vi "Save File DOE Get Program Info.vi"(10 "LV Program":T1=enum."DOE Stand", 11 "File Paths":T2={"General Setup Paths"={"Calibration File Path"=path "C:/Program Files/GE/Washer DOE/CalibrationDates.txt", "DOE Capacity Path"=path "C:/Program Files/GE/Washer DOE/DOE Capacity.txt", "Data Folder Path"=path "C:/Program Files/GE/Washer DOE/CalibrationDates.txt", "RLT Backup Data Path"=path "C:/Program Files/GE/Washer DOE/CalibrationDates.txt", "Tool Base Path"=path "C:/Program Files/GE/Washer DOE/CalibrationDates.txt", "General Startup Config Path"=path "C:/Program Files/GE/Washer DOE/CalibrationDates.txt", "File Save Previous Run Path"=path "", "File Save Configuration Data Path"=path ""}, "Data File Paths"={"Data File Path"=path "", "Debug File Path"=path "", "Bus Log Path"=path "", "Current"=path "", "Summary"=path ""}, "New Summary Created"=FALSE, "Check Location Interval (Second)"=0}) -> (1 "Headers":string[](array[string]), 2 "Model Information":string[][](array[string]), 3 "Program Names":string[](array[string]))   [LabVIEW 2016, in "File Setup.lvlib"]
uses:
  File Setup.lvlib
  File Setup (Public)/Type Definition/Save File DOE File Path Control.ctl
  File Setup (Public)/Type Definition/Save File DOE LabView Program.ctl
  File Setup (Public)/Type Definition/Save File DOE Data Save Filepaths.ctl
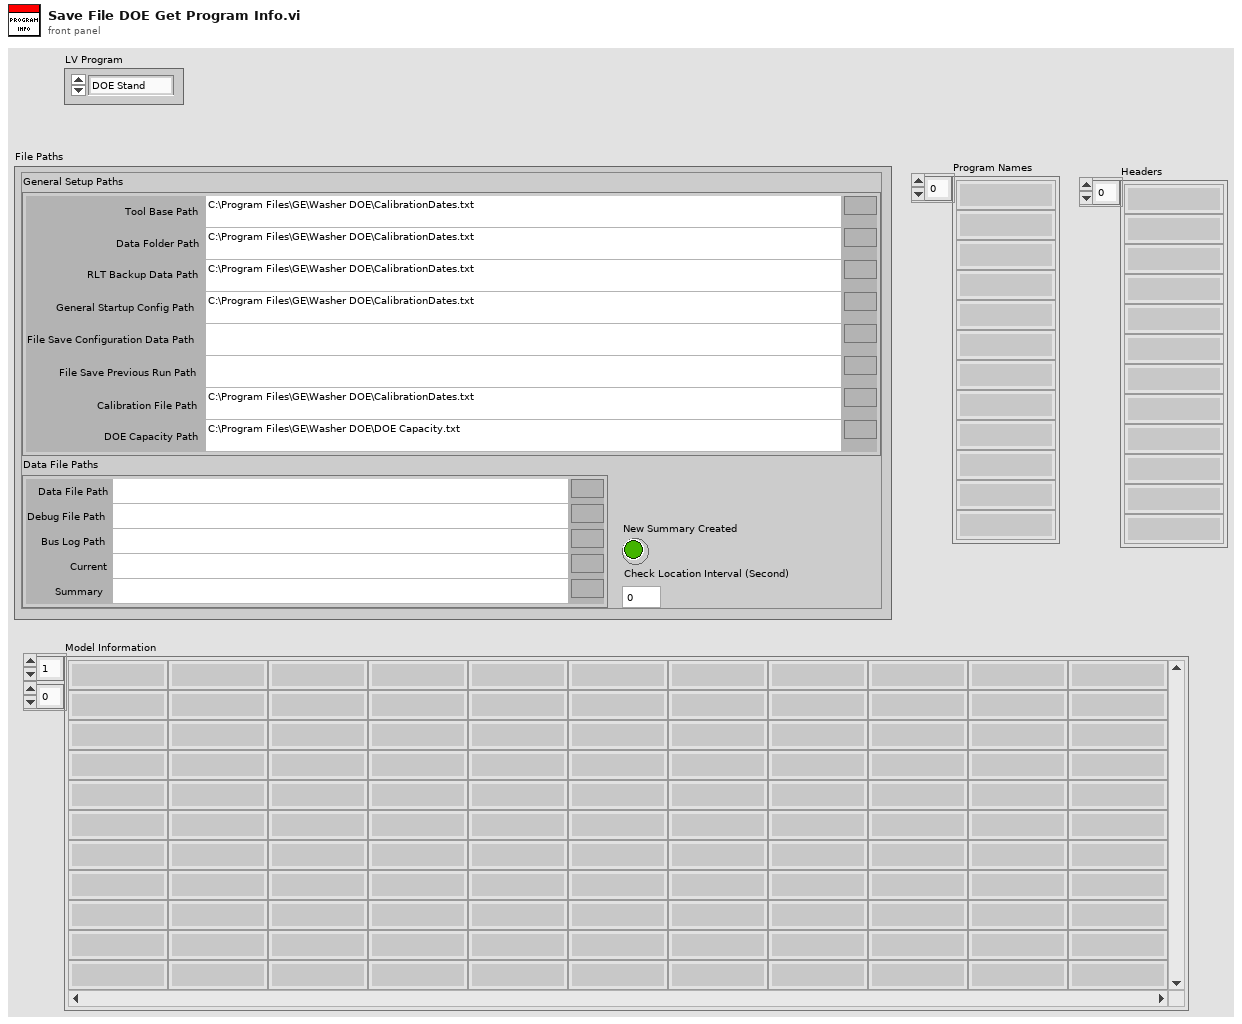
[diagram p1: front panel]
types:
  T1 = typedef "File Setup.lvlib/Save File DOE LabView Program.ctl" = enum16{"No Name Found", "DOE Stand", "Dishwasher Kitchen", "Portable Stand", "HEWH", "Dryer", "Dryer WILT", "HCC", "PRAT", "HEWH RLT"}
  T2 = typedef "File Setup.lvlib/Save File DOE File Path Control.ctl" = cluster{"General Setup Paths":cluster{"Calibration File Path":path, "DOE Capacity Path":path, "Data Folder Path":path, "RLT Backup Data Path":path, "Tool Base Path":path, "General Startup Config Path":path, "File Save Previous Run Path":path, "File Save Configuration Data Path":path}, "Data File Paths":T3, "New Summary Created":bool, "Check Location Interval (Second)":i32}
  T3 = typedef "File Setup.lvlib/Save File DOE Data Save Filepaths.ctl" = cluster{"Data File Path":path, "Debug File Path":path, "Bus Log Path":path, "Current":path, "Summary":path}
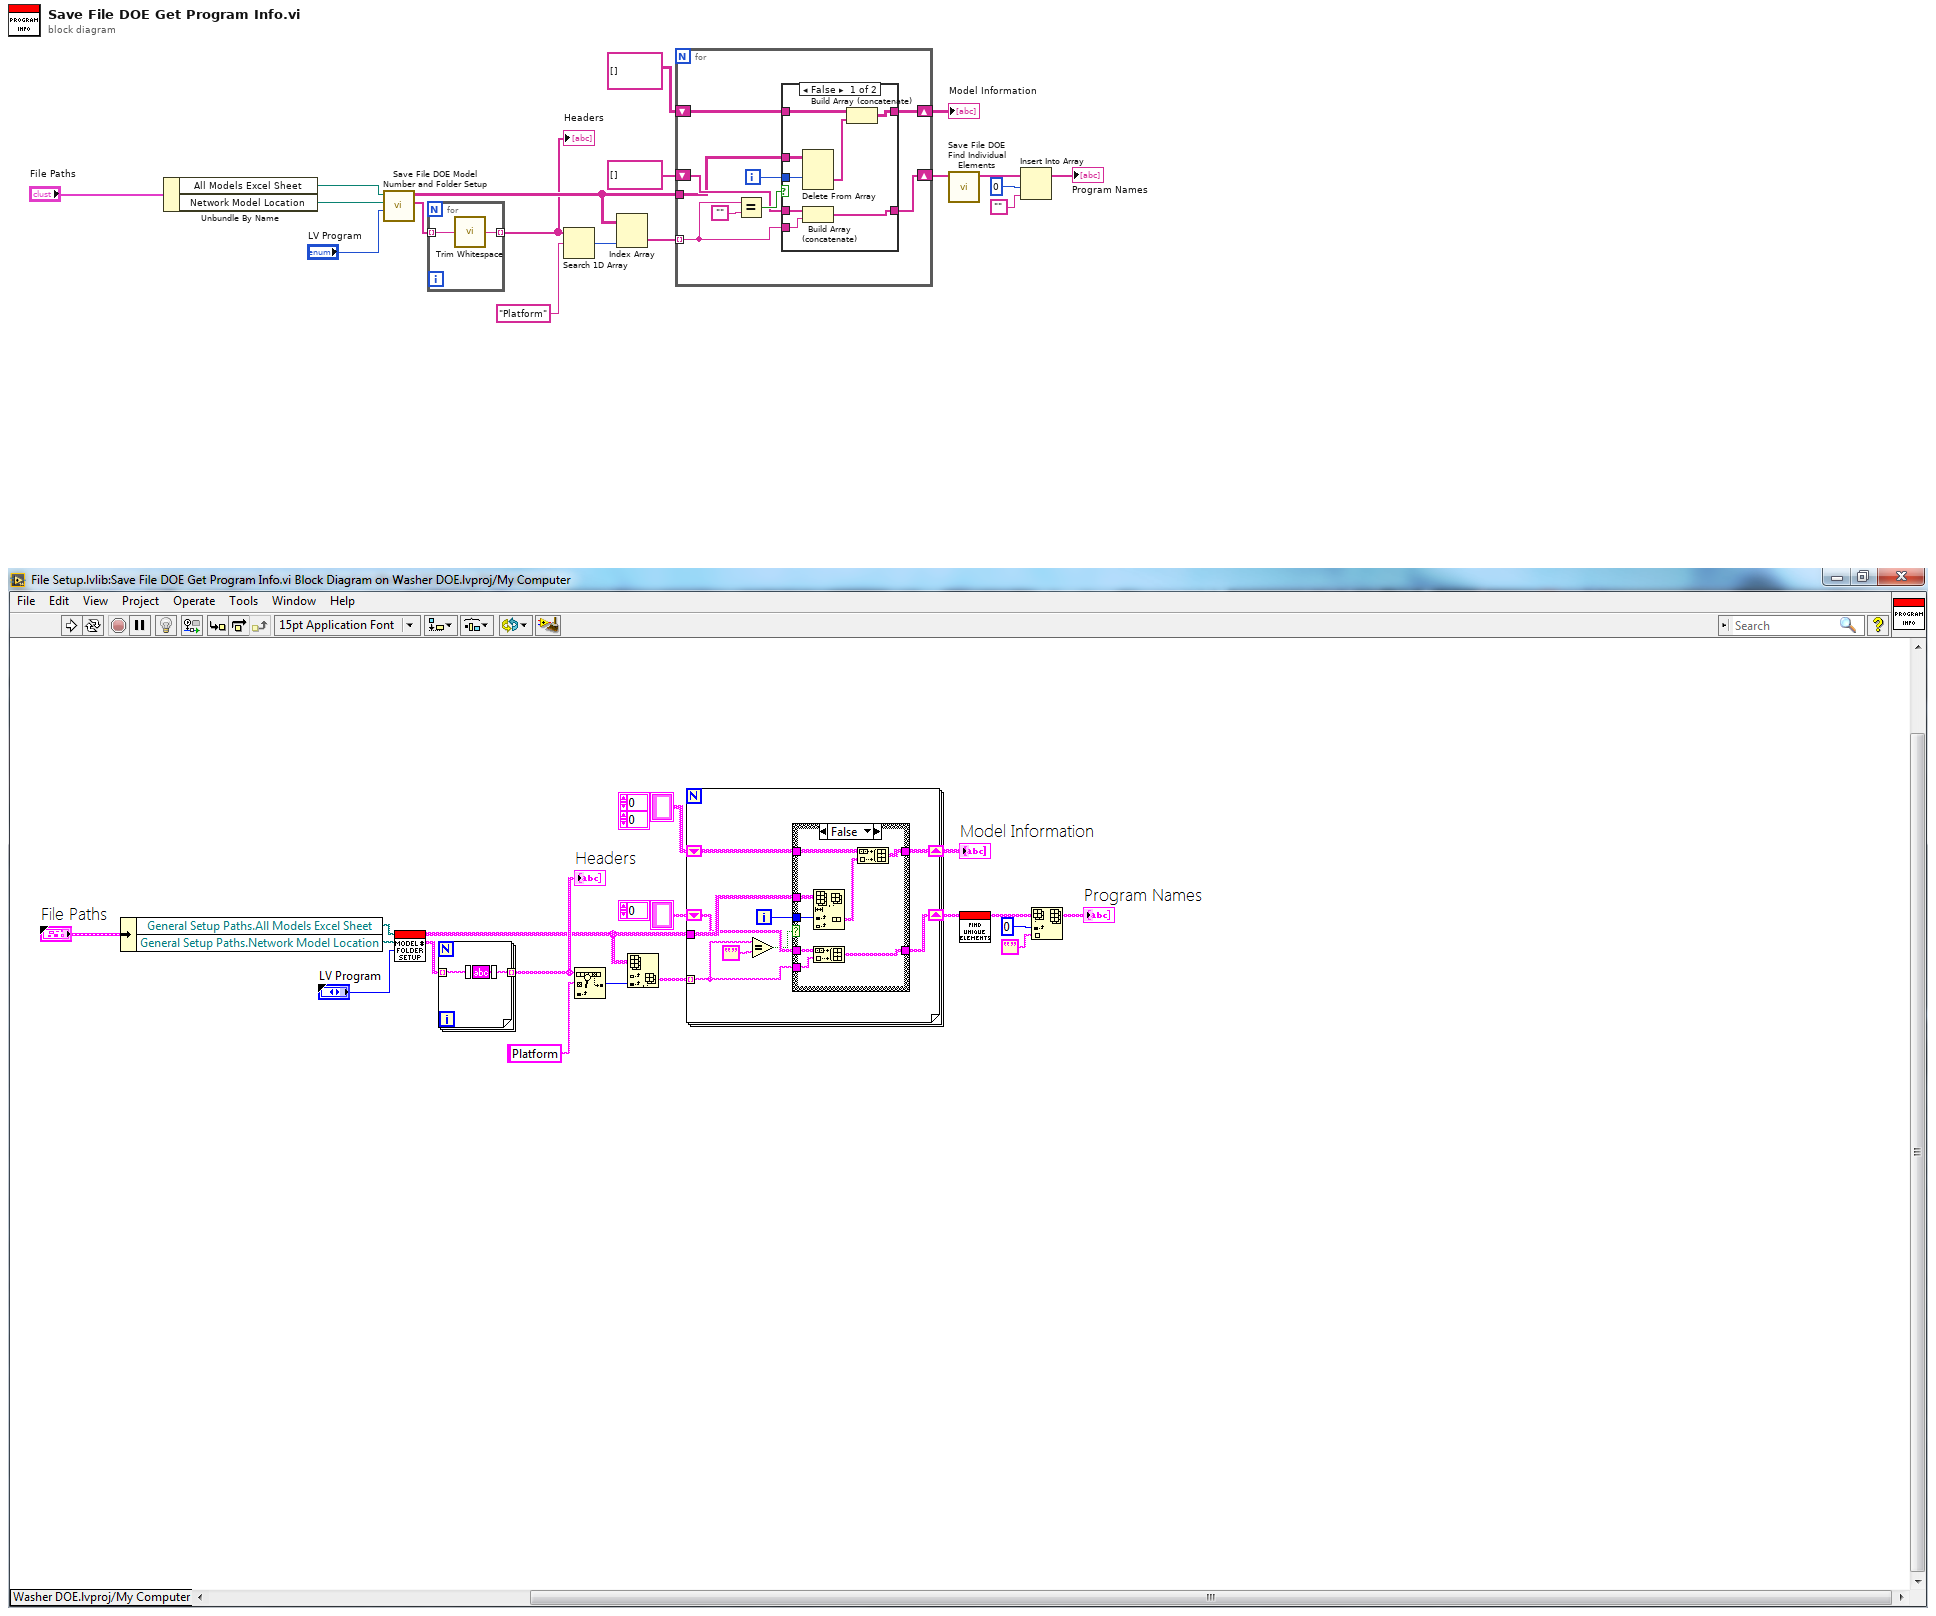
[diagram p0: block diagram]
diagram:
  n1 = Unbundle By Name("File Paths") -> ("All Models Excel Sheet"=w9:path, "Network Model Location"=w10:path)
  n2 = call "Save File DOE Model Number and Folder Setup.vi"("LV Program"="LV Program", "Network Model Location"=w10, "All Models Excel Sheet"=w9) -> ("Header"=w18:string[], "Model Data"=w15:string[][])  [unwired: 7 in]
  n3 = for {
    tunnel: w18 -> [w20] mode=indexing
    tunnel: [w19] -> w4 mode=indexing
    n4 = call <vilib>:"Trim Whitespace.vi"("string"=w20) -> ("trimmed string"=w19:string)  [unwired: 1 in]
  }
  "Headers" <- w4
  n5 = Search 1D Array(1D array=w4, element="Platform") -> (index of element=w2:i32)  [unwired: 1 in]
  n6 = Index Array(array=w15, index (col)=w2) -> (element=w12:string[])  [unwired: 1 in]
  n7 = for {
    tunnel: w12 -> [w26] mode=indexing
    shift-right: [w25] -> w14
    shift-left: string[] [] -> [w27]
    tunnel: w15 -> [w24]
    shift-right: [w21] -> w17
    shift-left: string[][] [] -> [w23]
    i -> [w22]
    n8 = Equal?(x=w26, y="") -> (x = y?=w28:bool)
    n9 = case shown="False" w28 {
      tunnel: w27 -> [w37 w39]
      tunnel: w26 -> [w36 _]
      tunnel: [w35 w39] -> w25
      tunnel: w24 -> [w34 _]
      tunnel: w23 -> [w33 w38]
      tunnel: w22 -> [w32 _]
      tunnel: [w30 w38] -> w21
      frame False {
        n10 = Delete From Array(array=w34, index (row)=w32) -> (deleted portion=w31:string[])  [unwired: 2 in, 1 out]
        n11 = Build Array (concatenate)(w37, w36) -> (w35:string[])
        n12 = Build Array (concatenate)(w33, w31) -> (w30:string[][])
      }
      frame True {
      }
    }
  }
  "Model Information" <- w17
  n13 = call "Save File DOE Find Individual Elements.vi"("Input Array"=w14) -> ("Individual Elements"=w8:string[])  [unwired: 10 in]
  n14 = Insert Into Array(array=w8, index=0, new element="") -> (→"Program Names":string[])
